vi "d2_encoder_test_ramp.vi"() -> ()   [LabVIEW 2014]
uses:
  <vilib>/eio/EIONode/EIONode.xnode
  <vilib>/rvi/FXPMathLib/FxpMul/XNode/nifxpmath_Multiplier.xnode
  <vilib>/rvi/FXPMathLib/sim/FxpSim.dll
  <vilib>/rvi/eio/common/nirviEmuTemplateMethod_errors.vi
  <vilib>/rvi/FXPMathLib/FxpSinAndCos/XNode/nifxpmath_SinAndCos.xnode
  <vilib>/rvi/FXPMathLib/FxpSinAndCos/simVIs/DllFxpSinAndCosTemp_sub.vi
  <vilib>/rvi/FXPMathLib/FxpSinAndCos/subVIs/nifxpmath_SinAndCos_SimConfig.ctl
  <vilib>/rvi/Analysis/measure/butterworth/XNode/niFpgaButterworthFilter.xnode
  <vilib>/rvi/FXPMathLib/FxpSub/XNode/nifxpmath_Sub.xnode
  <vilib>/rvi/FXPMathLib/FxpAdd/XNode/nifxpmath_Add.xnode
  <vilib>/rvi/DataTransferAndStorage/Container/XNode/niFpgaContainer.xnode
  <vilib>/rvi/interface/RandomDataEmulation/nirviRandomDataFpgaMultiElementTemplate.vi
panel:
  out "Dr":fxp<+/-,11,7>
  in  "D_end":fxp<+/-,11,7>
  in  "Command":i16(ring) items=["Step", "Ramp", "Sine"]
  out "D_i":fxp<+/-,34,18>
  in  "D_tolorence":fxp<+/-,14,3>
  in  "Ki":fxp<+/-,20,6>
  out "D_error":fxp<+/-,24,11>
  in  "Direction":bool
  out "Fmr_PD":fxp<+/-,64,31>
  in  "Kd":fxp<+/-,20,8>
  in  "Kp":fxp<+/-,20,12>
  in  "scaled coefficients_D_dd":i32[](array[numeric])=[780119100, 146811362]
  out "D_dd":fxp<+/-,36,29>
  in  "Ini coe.":bool
  out "va":fxp<+/-,38,8>
  out "vb":fxp<+/-,38,8>
  in  "stop motor":bool
  out "vq_F":fxp<+/-,20,5> format="%.57g"
  out "vd_F":fxp<+/-,20,5>
  out "D_d (mm/s)":fxp<+/-,32,12>
  out "mt":u32
  out "omega (rad/s)":fxp<+/-,32,18>
  in  "mt0":u32
  out "D(mm)":fxp<+/-,22,7>
  out "rad(NrTheta)":fxp<+/-,33,18>
  out "Encoder Position":i32
  in  "Encoder Reset":bool
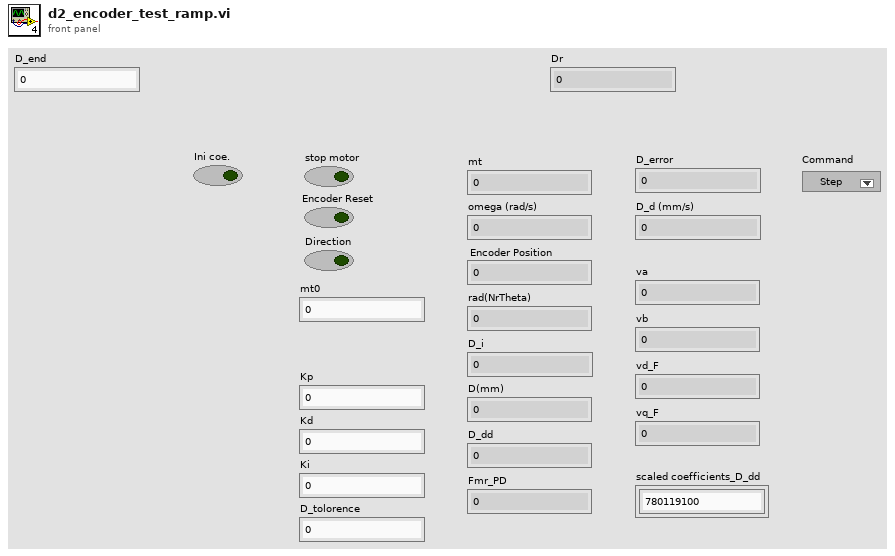
[diagram p1: front panel]
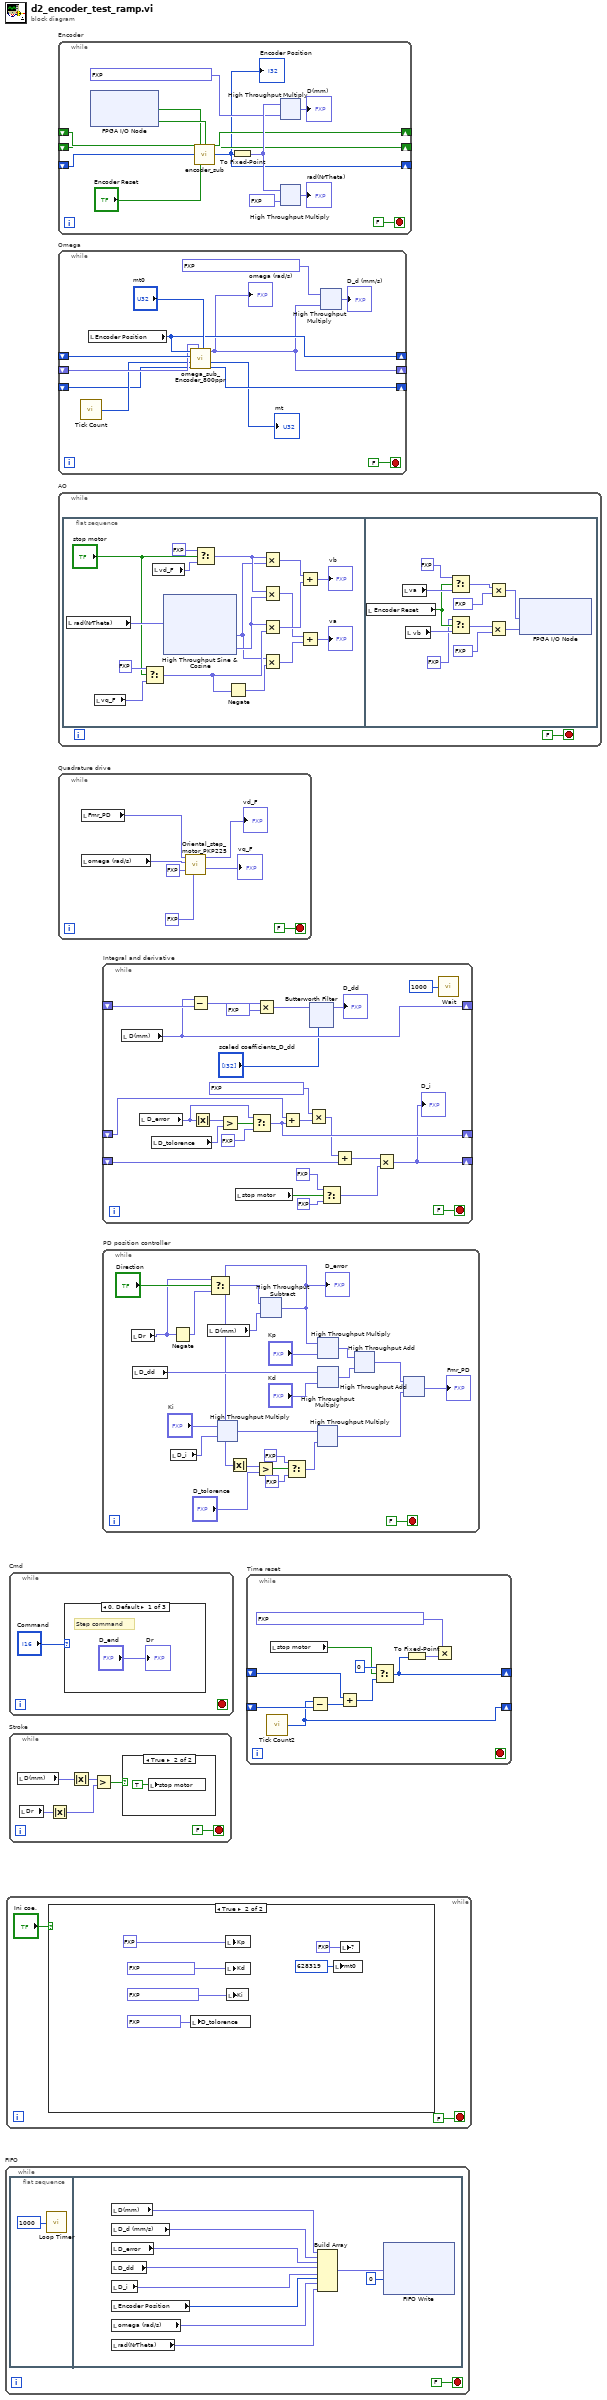
[diagram p0: block diagram]
diagram:
  n1 = while "FIFO" {
    stop <- FALSE stop-if-true
    n2 = flat-sequence {
      frame #0 {
        n3 = call "Loop Timer"("Count(uSec)"=u32 1000) -> ()  [unwired: 1 out]
      }
      frame #1 {
        n4 = local read "D(mm)"() -> (w10:fxp<+/-,22,7>)
        n5 = local read "D_d (mm/s)"() -> (w9:fxp<+/-,32,12>)
        n6 = local read "D_error"() -> (w8:fxp<+/-,24,11>)
        n7 = local read "D_dd"() -> (w7:fxp<+/-,36,29>)
        n8 = local read "D_i"() -> (w6:fxp<+/-,34,18>)
        n9 = local read "Encoder Position"() -> (w5:i32)
        n10 = local read "omega (rad/s)"() -> (w4:fxp<+/-,32,18>)
        n11 = local read "rad(NrTheta)"() -> (w3:fxp<+/-,33,18>)
        n12 = Build Array(w10, w9, w8, w7, w6, w5, w4, w3) -> (w11:fxp<+/-,52,32>[])
        n13 = xnode ("FIFO Write")("Element"=w11, "Timeout"=0) -> ()  [unwired: 1 in, 2 out]
      }
    }
  }
  n14 = while {
    stop <- FALSE stop-if-true
    n15 = case shown="True" "Ini coe." {
      frame False {
      }
      frame True {
        n16 = local write "D_tolorence"(fxp<+/-,14,3> 0.009765625 ("D_tolorence")) -> ()
        n17 = local write "Kp"(fxp<+/-,20,12> 2.0 ("Kp")) -> ()
        n18 = local write "Kd"(fxp<+/-,20,8> 1.800048828125 ("Kd")) -> ()
        n19 = local write "Ki"(fxp<+/-,20,6> 0.0999755859375 ("D_i")) -> ()
        n20 = local write "mt0"(u32 628319 ("mt0")) -> ()
        n21 = local write item#-1(fxp<+/-,11,7> 20.0 ("Fmr")) -> ()
      }
    }
  }
  n22 = while "Cmd" {
    stop <- _ stop-if-true
    n23 = case shown="0, Default" "Command" {
      frame 0, Default {
        # "Step command"
        "Dr" <- "D_end"
      }
      frame 1 {
      }
      frame 2 {
      }
    }
  }
  n24 = while "Stroke" {
    stop <- FALSE stop-if-true
    n25 = local read "D(mm)"() -> (w28:fxp<+/-,22,7>)
    n26 = local read "Dr"() -> (w24:fxp<+/-,11,7>)
    n27 = Absolute Value(x=w24) -> (abs(x)=w23:fxp<+,11,7>)
    n28 = Absolute Value(x=w28) -> (abs(x)=w27:fxp<+,22,7>)
    n29 = Greater?(x=w27, y=w23) -> (0:w26:bool)
    n30 = case shown="True" w26 {
      frame False {
      }
      frame True {
        n31 = local write "stop motor"(TRUE ("stop motor")) -> ()
      }
    }
  }
  n32 = while "Encoder" {
    shift-right: [w36] -> _
    shift-left: _ -> [w38]
    shift-right: [w35] -> _
    shift-left: _ -> [w37]
    shift-right: [w33] -> _
    shift-left: _ -> [w34]
    stop <- FALSE stop-if-true
    n33 = xnode "FPGA I/O Node"() -> ("Mod4/DI3"=w43:bool, "Mod4/DI4"=w44:bool)  [unwired: 2 in, 2 out]
    n34 = call "encoder_sub.vi"("A_pre"=w38, "B_pre"=w37, "Encoder Position_pre"=w34, "A input"=w43, "Encoder Position Reset"="Encoder Reset", "B input"=w44) -> ("A"=w36:bool, "B"=w35:bool, "Encoder Position (Counts)"=w33:i32)  [unwired: 19 in]
    "Encoder Position" <- w33
    n35 = To Fixed-Point(number=w33) -> (fixed-point=w41:fxp<+/-,32,32>)  [unwired: 1 in]
    n36 = xnode ("High Throughput Multiply")("x"=w41, "y"=fxp<+/-,24,0> 0.002499997615814209) -> ("x*y"=→"D(mm)":fxp<+/-,56,32>)
    n37 = xnode ("High Throughput Multiply")("x"=w41, "y"=fxp<+/-,24,0> 0.125) -> ("x*y"=→"rad(NrTheta)":fxp<+/-,56,32>)
  }
  n38 = while "Omega" {
    shift-right: [w54] -> _
    shift-left: _ -> [w55]
    shift-right: [w47] -> _
    shift-left: _ -> [w53]
    shift-right: [w50] -> _
    shift-left: _ -> [w51]
    stop <- FALSE stop-if-true
    n39 = call "Tick Count"() -> ("Tick Count(Ticks)"=w52:u32)
    n40 = local read "Encoder Position"() -> (w54:i32)
    n41 = call "omega_sub_Encoder_800ppr.vi"("mt0"="mt0", "omega_pre"=w53, "ticks_m_pre"=w51, "ticks"=w52, "count_pre"=w55, "count"=w54) -> ("ticks_m"=w50:u32, "mt"=→"mt":u32, "omega"=w47:fxp<+/-,20,9>)  [unwired: 3 in]
    "omega (rad/s)" <- w47
    n42 = xnode ("High Throughput Multiply")("x"=fxp<+/-,26,1> 0.3183099031448364, "y"=w47) -> ("x*y"=→"D_d (mm/s)":fxp<+/-,46,10>)
  }
  n43 = while "AO" {
    stop <- FALSE stop-if-true
    n44 = flat-sequence {
      frame #0 {
        n45 = local read "rad(NrTheta)"() -> (w73:fxp<+/-,33,18>)
        n46 = local read "vq_F"() -> (w71:fxp<+/-,20,5>)
        n47 = Select(t=fxp<+,20,5> 0.0, s="stop motor", f=w71) -> (s? t:f=w68:fxp<+/-,21,6>)
        n48 = local read "vd_F"() -> (w72:fxp<+/-,20,5>)
        n49 = xnode "High Throughput Sine & Cosine"("x (pi)"=w73) -> ("sin(x)"=w64:fxp<+/-,17,2>, "cos(x)"=w66:fxp<+/-,17,2>)
        n50 = Select(t=fxp<+,20,5> 0.0, s="stop motor", f=w72) -> (s? t:f=w65:fxp<+/-,21,6>)
        n51 = Negate(x=w68) -> (-x=w67:fxp<+/-,21,6>)
        n52 = Multiply(x=w65, y=w64) -> (x*y=w63:fxp<+/-,37,7>)
        n53 = Multiply(x=w65, y=w66) -> (x*y=w61:fxp<+/-,37,7>)
        n54 = Multiply(x=w66, y=w68) -> (x*y=w62:fxp<+/-,37,7>)
        n55 = Multiply(x=w64, y=w67) -> (x*y=w60:fxp<+/-,37,7>)
        n56 = Add(x=w63, y=w62) -> (x+y=→"vb":fxp<+/-,38,8>)
        n57 = Add(x=w61, y=w60) -> (x+y=→"va":fxp<+/-,38,8>)
      }
      frame #1 {
        n58 = local read "Encoder Reset"() -> (w107:bool)
        n59 = local read "va"() -> (w109:fxp<+/-,38,8>)
        n60 = local read "vb"() -> (w108:fxp<+/-,38,8>)
        n61 = Select(t=fxp<+/-,20,5> 5.0 ("y"), s=w107, f=w109) -> (s? t:f=w110:fxp<+/-,38,8>)
        n62 = Select(t=fxp<+/-,20,5> 0.0 ("y"), s=w107, f=w108) -> (s? t:f=w111:fxp<+/-,38,8>)
        n63 = Multiply(x=w111, y=fxp<+/-,20,5> -0.5) -> (x*y=w115:fxp<+/-,57,12>)
        n64 = Multiply(x=w110, y=fxp<+/-,20,5> -0.5) -> (x*y=w114:fxp<+/-,57,12>)
        n65 = xnode "FPGA I/O Node"("Mod8/AO0"=w114, "Mod8/AO1"=w115) -> ()  [unwired: 2 in, 2 out]
      }
    }
  }
  n66 = while "Quadrature drive" {
    stop <- FALSE stop-if-true
    n67 = local read "Fmr_PD"() -> (w116:fxp<+/-,64,31>)
    n68 = local read "omega (rad/s)"() -> (w118:fxp<+/-,32,18>)
    n69 = call "Oriental_step_motor_PKP225.vi"("F_Threshold"=fxp<+,12,12> 10.0, "dFmr"=fxp<+/-,25,15> 0.0, "omega"=w118, "Fmr"=w116) -> ("vq_F"=→"vq_F":fxp<+/-,20,5>, "vd_F"=→"vd_F":fxp<+/-,20,5>)  [unwired: 6 in]
  }
  n70 = while "Integral and derivative" {
    shift-right: [w143] -> _
    shift-left: _ -> [w147]
    shift-right: [w133] -> _
    shift-left: _ -> [w134]
    shift-right: [w123] -> _
    shift-left: _ -> [w127]
    stop <- FALSE stop-if-true
    n71 = local read "D(mm)"() -> (w143:fxp<+/-,22,7>)
    n72 = local read "D_error"() -> (w135:fxp<+/-,24,11>)
    n73 = local read "D_tolorence"() -> (w138:fxp<+/-,14,3>)
    n74 = Subtract(x=w143, y=w147) -> (x-y=w146:fxp<+/-,23,8>)
    n75 = Absolute Value(x=w135) -> (abs(x)=w139:fxp<+,24,11>)
    n76 = Greater?(x=w139, y=w138) -> (0:w137:bool)
    n77 = local read "stop motor"() -> (w130:bool)
    n78 = Select(t=w135, s=w137, f=fxp<+,24,11> 0.0) -> (s? t:f=w133:fxp<+/-,25,12>)
    n79 = Multiply(x=w146, y=fxp<+/-,33,13> 1000.0) -> (x*y=w144:fxp<+/-,55,20>)
    n80 = Add(x=w134, y=w133) -> (x+y=w132:fxp<+/-,26,13>)
    n81 = Multiply(x=fxp<+/-,30,12> 0.000499725341796875, y=w132) -> (x*y=w126:fxp<+/-,55,24>)
    n82 = xnode "Butterworth Filter"("input data"=w144, "scaled coefficients"="scaled coefficients_D_dd") -> ("output data"=→"D_dd":fxp<+/-,36,24>)  [unwired: 1 in]
    n83 = Select(t=fxp<+,1,1> 0.0, s=w130, f=fxp<+,1,1> 1.0) -> (s? t:f=w124:fxp<+,1,1>)
    n84 = Add(x=w126, y=w127) -> (x+y=w125:fxp<+/-,32,16>)
    n85 = Multiply(x=w125, y=w124) -> (x*y=w123:fxp<+/-,32,16>)
    "D_i" <- w123
    n86 = call "Wait"("Count(uSec)"=u32 1000) -> ()  [unwired: 1 out]
  }
  n87 = while "PD position controller" {
    stop <- FALSE stop-if-true
    n88 = local read "Dr"() -> (w157:fxp<+/-,11,7>)
    n89 = local read "D_dd"() -> (w176:fxp<+/-,36,29>)
    n90 = local read "D_i"() -> (w168:fxp<+/-,34,18>)
    n91 = Negate(x=w157) -> (-x=w172:fxp<+/-,12,8>)
    n92 = local read "D(mm)"() -> (w180:fxp<+/-,22,7>)
    n93 = Select(t=w157, s="Direction", f=w172) -> (s? t:f=w171:fxp<+/-,12,8>)
    n94 = xnode ("High Throughput Multiply")("x"="Ki", "y"=w168) -> ("x*y"=w162:fxp<+/-,54,24>)
    n95 = xnode "High Throughput Subtract"("x"=w171, "y"=w180) -> ("x-y"=w166:fxp<+/-,24,9>)
    "D_error" <- w166
    n96 = Absolute Value(x=w166) -> (abs(x)=w167:fxp<+,24,9>)
    n97 = Greater?(x=w167, y="D_tolorence") -> (0:w165:bool)
    n98 = Select(t=fxp<+,10,2> 1.0, s=w165, f=fxp<+,10,2> 0.0) -> (s? t:f=w161:fxp<+,10,2>)
    n99 = xnode ("High Throughput Multiply")("x"=w162, "y"=w161) -> ("x*y"=w158:fxp<+/-,64,26>)
    n100 = xnode ("High Throughput Multiply")("x"=w166, "y"="Kp") -> ("x*y"=w178:fxp<+/-,44,21>)
    n101 = xnode ("High Throughput Multiply")("x"=w176, "y"="Kd") -> ("x*y"=w177:fxp<+/-,56,37>)
    n102 = xnode ("High Throughput Add")("x"=w178, "y"=w177) -> ("x+y"=w159:fxp<+/-,61,38>)
    n103 = xnode ("High Throughput Add")("x"=w159, "y"=w158) -> ("x+y"=→"Fmr_PD":fxp<+/-,64,39>)
  }
  n104 = while "Time reset" {
    shift-right: [w183] -> _
    shift-left: _ -> [w187]
    shift-right: [w188] -> _
    shift-left: _ -> [w189]
    stop <- _ stop-if-true
    n105 = call "Tick Count2"() -> ("Tick Count(uSec)"=w188:u32)
    n106 = local read "stop motor"() -> (w184:bool)
    n107 = Subtract(x=w188, y=w189) -> (x-y=w190:u32)
    n108 = Add(x=w187, y=w190) -> (x+y=w186:u32)
    n109 = Select(t=u32 0, s=w184, f=w186) -> (s? t:f=w183:u32)
    n110 = To Fixed-Point(number=w183) -> (fixed-point=w182:fxp<+,32,32>)  [unwired: 1 in]
    n111 = Multiply(x=fxp<+,20,-18> 1.0000003385357559e-06, y=w182) -> ()  [unwired: 1 out]
  }
